vi "Zaber A Series IO Ports.vi"() -> ()   [LabVIEW 2018]
doc: "This example shows how you can query and set inputs and outputs when they are available on Zaber controllers, such as the A-MCB2, X-MCB1, and X-MCB2. This example will not function when connected to a device that does not have I/O ports."
uses:
  Zaber A Series.lvlib
panel:
  out "Analog Output 4":dbl
  out "Analog Output 3":dbl
  out "Analog Output 2":dbl
  in  "Analog Out 4 (Volts)":dbl
  in  "Analog Out 3 (Volts)":dbl
  in  "Analog Out 2 (Volts)":dbl
  out "Analog Output 1":dbl
  in  "Analog Out 1 (Volts)":dbl
  out "Analog Output Count":i32
  out "Digital Output Count":i32
  out "Digital Input Count":i32
  out "Analog Input Count":i32
  in  "Device Number":string
  out "Digital Output 4":bool
  out "Digital Output 3":bool
  out "Digital Output 2":bool
  out "Digital Output 1":bool
  out "Analog In 4 (Volts)":string
  out "Analog In 3 (Volts)":string
  out "Analog In 2 (Volts)":string
  out "Analog In 1 (Volts)":string
  out "Digital In 4":bool
  out "Digital In 3":bool
  out "Digital In 2":bool
  out "Digital In 1":bool
  in  "Digital Out 4":bool
  in  "Digital Out 3":bool
  in  "Digital Out 2":bool
  in  "Digital Out 1":bool
  in  "VISA resource name":refnum<visa-resource-name>
  out "Port Open":bool
  in  "Quit":bool
  in  "Open Port":bool
  in  "Close Port":bool
  # "(c) 2017-2020 Zaber Technologies.  ALL RIGHTS RESERVED."
  # "Some Zaber devices, including the A-MCB, X-MCB and X-MCC series controllers have inputs and outputs. This example shows how you can read and parse these inputs. Once the port is open, it will poll the IOs and update the information. You can easily switch the digital outputs to update them as well."
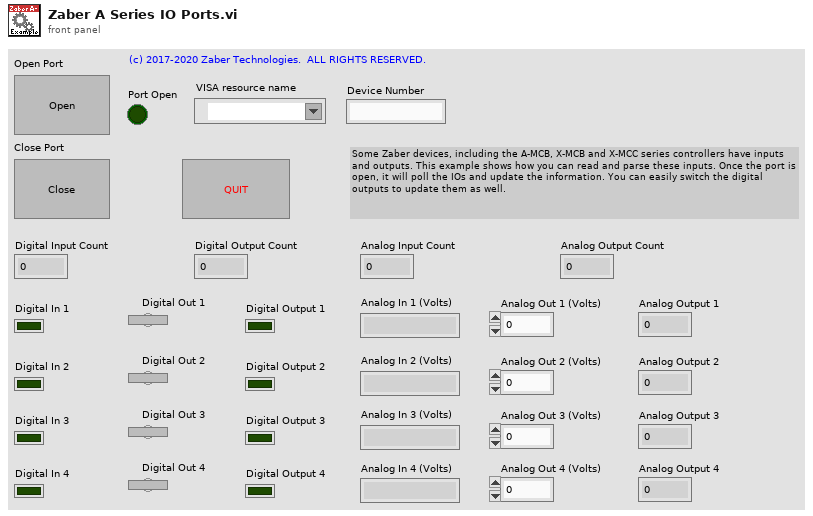
[diagram p1: front panel]
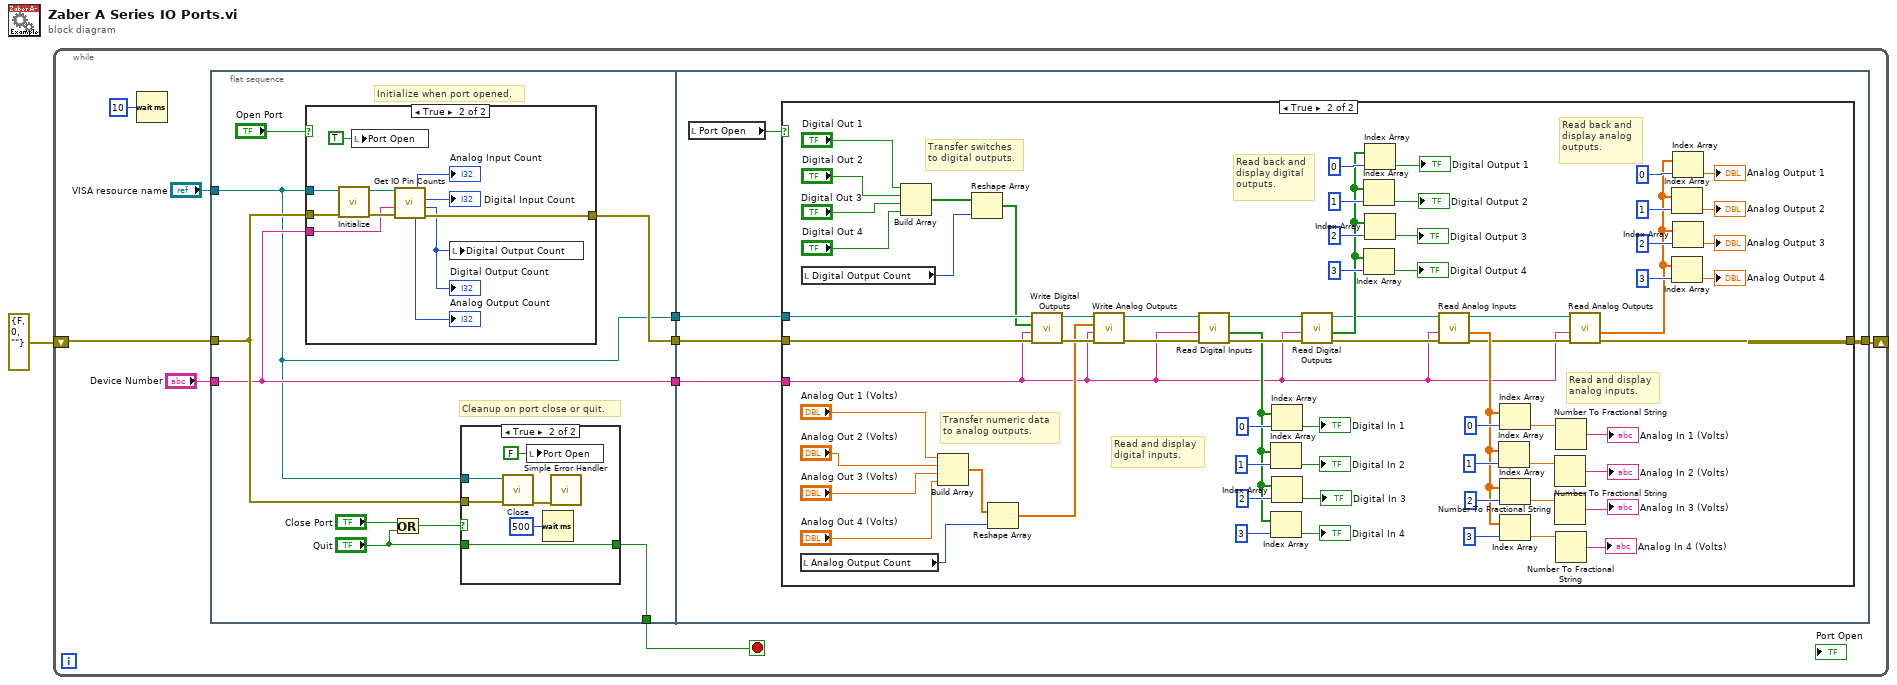
[diagram p0: block diagram]
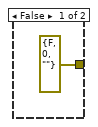
[diagram p3: hidden frame]
diagram:
  n1 = while {
    shift-right: [w2] -> _
    shift-left: errorcluster {"status"=FALSE, "code"=0, "source"=""} ("error out") -> [w6]
    stop <- w9 stop-if-true
    n2 = Wait (ms)(milliseconds to wait=u32 10) -> ()  [unwired: 1 out]
    n3 = flat-sequence {
      tunnel: "VISA resource name" -> [w11]
      tunnel: [w11] -> w10
      tunnel: [w15] -> w9
      tunnel: [w14] -> w7
      tunnel: w6 -> [w13]
      tunnel: "Device Number" -> [w12]
      tunnel: [w12] -> w3
      tunnel: w10 -> [w40]
      tunnel: w7 -> [w43]
      tunnel: [w42] -> w2
      tunnel: w3 -> [w41]
      frame #0 {
        # "Cleanup on port close or quit."
        # "Initialize when port opened."
        n4 = case shown="True" "Open Port" {
          tunnel: w11 -> [_ w38]
          tunnel: [errorcluster {"status"=FALSE, "code"=0, "source"=""} ("error in (no error)") w33] -> w14
          tunnel: w13 -> [_ w36]
          tunnel: w12 -> [_ w28]
          frame False {
          }
          frame True {
            n5 = call "Initialize.vi"("error in (no error)"=w36, "VISA resource name"=w38) -> ("error out"=w35:errorcluster, "VISA resource name out"=w34:refnum<visa-resource-name>)  [unwired: 8 in]
            n6 = local write "Port Open"(TRUE) -> ()
            n7 = call "Get IO Pin Counts.vi"("error in (no error)"=w35, "Device Number"=w28, "VISA resource name"=w34) -> ("error out"=w33:errorcluster, "Digital Output Count"=w29:i32, "Digital Input Count"=→"Digital Input Count":i32, "Analog Output Count"=→"Analog Output Count":i32, "Analog Input Count"=→"Analog Input Count":i32)  [unwired: 3 in, 1 out]
            "Digital Output Count" <- w29
            n8 = local write "Digital Output Count"(w29) -> ()
          }
        }
        n9 = Or(x="Close Port", y="Quit") -> (x .or. y?=w18:bool)
        n10 = case shown="True" w18 {
          tunnel: w11 -> [_ w24]
          tunnel: [w20 w26] -> w15
          tunnel: "Quit" -> [w20 w26]
          tunnel: w13 -> [_ w23]
          frame False {
          }
          frame True {
            n11 = call "Close.vi"("error in (no error)"=w23, "VISA resource name"=w24) -> ("error out"=w22:errorcluster)  [unwired: 9 in]
            n12 = local write "Port Open"(FALSE) -> ()
            n13 = Wait (ms)(milliseconds to wait=u32 500) -> ()  [unwired: 1 out]
            n14 = call <vilib>:"Simple Error Handler.vi"("error in (no error)"=w22) -> ()  [unwired: 4 in, 5 out]
          }
        }
      }
      frame #1 {
        n15 = local read "Port Open"() -> (w39:bool)
        n16 = case shown="True" w39 {
          tunnel: w40 -> [_ w80]
          tunnel: w43 -> [w44 w81]
          tunnel: [w44 w56] -> w42
          tunnel: w41 -> [_ w54]
          frame False {
          }
          frame True {
            # "Read back and\ndisplay analog \noutputs."
            # "Transfer numeric data\nto analog outputs."
            # "Read and display\nanalog inputs."
            # "Read and display\ndigital inputs."
            # "Read back and\ndisplay digital \noutputs."
            # "Transfer switches\nto digital outputs."
            n17 = local read "Analog Output Count"() -> (w62:i32)
            n18 = local read "Digital Output Count"() -> (w74:i32)
            n19 = Build Array("Digital Out 1", "Digital Out 2", "Digital Out 3", "Digital Out 4") -> (w75:bool[])
            n20 = Build Array("Analog Out 1 (Volts)", "Analog Out 2 (Volts)", "Analog Out 3 (Volts)", "Analog Out 4 (Volts)") -> (w63:dbl[])
            n21 = Reshape Array(w75, w74) -> (w68:bool[])
            n22 = Reshape Array(w63, w62) -> (w57:dbl[])
            n23 = call "Write Digital Outputs.vi"("error in (no error)"=w81, "Device Number"=w54, "Digital Outputs"=w68, "VISA resource name"=w80) -> ("error out"=w59:errorcluster, "VISA resource name out"=w61:refnum<visa-resource-name>)  [unwired: 6 in]
            n24 = call "Write Analog Outputs.vi"("error in (no error)"=w59, "Device Number"=w54, "Analog Outputs"=w57, "VISA resource name"=w61) -> ("error out"=w58:errorcluster, "VISA resource name out"=w60:refnum<visa-resource-name>)  [unwired: 6 in]
            n25 = call "Read Digital Inputs.vi"("error in (no error)"=w58, "Device Number"=w54, "VISA resource name"=w60) -> ("error out"=w72:errorcluster, "Digital Input Pins"=w69:bool[], "VISA resource name out"=w73:refnum<visa-resource-name>)  [unwired: 6 in]
            n26 = Index Array(array=w69, index=1) -> (element=→"Digital In 2":bool)
            n27 = Index Array(array=w69, index=3) -> (element=→"Digital In 4":bool)
            n28 = Index Array(array=w69, index=0) -> (element=→"Digital In 1":bool)
            n29 = Index Array(array=w69, index=2) -> (element=→"Digital In 3":bool)
            n30 = call "Read Digital Outputs.vi"("error in (no error)"=w72, "Device Number"=w54, "VISA resource name"=w73) -> ("error out"=w71:errorcluster, "Digital Output Pins"=w86:bool[], "VISA resource name out"=w70:refnum<visa-resource-name>)  [unwired: 6 in]
            n31 = Index Array(array=w86, index=1) -> (element=→"Digital Output 2":bool)
            n32 = Index Array(array=w86, index=3) -> (element=→"Digital Output 4":bool)
            n33 = Index Array(array=w86, index=0) -> (element=→"Digital Output 1":bool)
            n34 = Index Array(array=w86, index=2) -> (element=→"Digital Output 3":bool)
            n35 = call "Read Analog Inputs.vi"("error in (no error)"=w71, "Device Number"=w54, "VISA resource name"=w70) -> ("error out"=w56:errorcluster, "Analog Inputs"=w99:dbl[], "VISA resource name out"=w55:refnum<visa-resource-name>)  [unwired: 6 in]
            n36 = Index Array(array=w99, index=1) -> (element=w96:dbl)
            n37 = Index Array(array=w99, index=0) -> (element=w97:dbl)
            n38 = Index Array(array=w99, index=2) -> (element=w93:dbl)
            n39 = Index Array(array=w99, index=3) -> (element=w91:dbl)
            n40 = Number To Fractional String(number=w96) -> (F-format string=→"Analog In 2 (Volts)":string)  [unwired: 3 in]
            n41 = Number To Fractional String(number=w93) -> (F-format string=→"Analog In 3 (Volts)":string)  [unwired: 3 in]
            n42 = Number To Fractional String(number=w97) -> (F-format string=→"Analog In 1 (Volts)":string)  [unwired: 3 in]
            n43 = Number To Fractional String(number=w91) -> (F-format string=→"Analog In 4 (Volts)":string)  [unwired: 3 in]
            n44 = call "Read Analog Outputs.vi"("error in (no error)"=w56, "Device Number"=w54, "VISA resource name"=w55) -> ("Analog Outputs"=w49:dbl[])  [unwired: 6 in, 2 out]
            n45 = Index Array(array=w49, index=1) -> (element=→"Analog Output 2":dbl)
            n46 = Index Array(array=w49, index=3) -> (element=→"Analog Output 4":dbl)
            n47 = Index Array(array=w49, index=0) -> (element=→"Analog Output 1":dbl)
            n48 = Index Array(array=w49, index=2) -> (element=→"Analog Output 3":dbl)
          }
        }
      }
    }
  }
